vi "ReadSingleCANFrame.vi"(8 "error in (no error)":errorcluster, 11 "BLF File In":refnum<class "Read Write BLF.lvclass">) -> (0 "error out":errorcluster, 1 "CAN Channel":u16, 2 "CAN Frame":T1 {"type" items=["CAN Data"=0, "CAN Remote"=1, "CAN Bus Error"=2, "CAN 2.0 Data"=8, "CAN FD Data"=16, "CAN FD+BRS Data"=24, "J1939 Data"=192, "Delay"=224, "Log Trigger"=225, "Start Trigger"=226]; "payload" format="%x"; "timestamp" format="%<%.7X\n%x>T"; "identifier" format="%x"}, 3 "BLF File Out":refnum<class "Read Write BLF.lvclass">)   [LabVIEW 2015, in "Read Write BLF.lvclass"]
doc: "This VI will read <B>CAN Frames</B> from a BLF file. Optionally enter the <B>Offset</B> and <B>Length</B> which defaults to all. This will read the set number of Objects which might not correspond to the same number of frames.\n\n-------------\nBrian Hoover (Hooovahh)"
uses:
  Read Write BLF.lvclass
  Controls/Cluster - CAN Frame.ctl
  Controls/Enum - CAN Data Type.ctl
  Controls/Enum - Read Object Types.ctl
  Read Write BLF.lvclass/Read Write BLF.ctl
  SubVIs/GetBinlogdllpath.vi
  <vilib>/Utility/error.llb/Error Cluster From Error Code.vi
  <vilib>/Utility/libraryn.llb/Check if File or Folder Exists.vi
  <vilib>/Utility/file.llb/Application Directory.vi
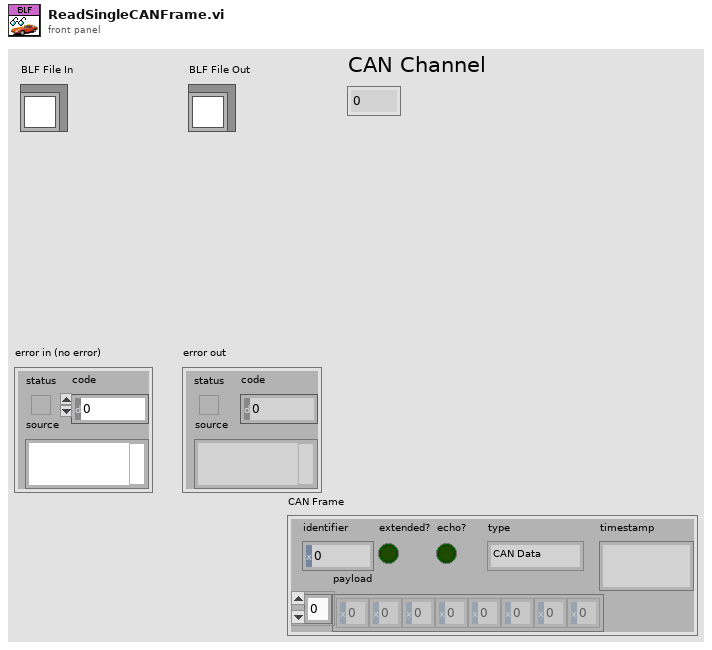
[diagram p1: front panel]
types:
  T1 = typedef "Read Write BLF.lvclass/Cluster - CAN Frame.ctl" = cluster{"timestamp":timestamp, "payload":u8[], "identifier":u32, "extended?":bool, "echo?":bool, "type":T2}
  T2 = typedef "Read Write BLF.lvclass/Enum - CAN Data Type.ctl" = u8
  T3 = typedef "Read Write BLF.lvclass/Enum - Read Object Types.ctl" = enum32{"UNKNOWN", "CAN_MESSAGE", "CAN_ERROR", "CAN_OVERLOAD", "CAN_STATISTIC", "APP_TRIGGER", "ENV_INTEGER", "ENV_DOUBLE", "ENV_STRING", "ENV_DATA", "LOG_CONTAINER", "LIN_MESSAGE", "LIN_CRC_ERROR", "LIN_DLC_INFO", "LIN_RCV_ERROR", "LIN_SND_ERROR", "LIN_SLV_TIMEOUT", "LIN_SCHED_MODCH", "LIN_SYN_ERROR", "LIN_BAUDRATE", "LIN_SLEEP", "LIN_WAKEUP", "MOST_SPY", "MOST_CTRL", "MOST_LIGHTLOCK", "MOST_STATISTIC", "reserved_1", "reserved_2", "reserved_3", "FLEXRAY_DATA", "FLEXRAY_SYNC", "CAN_DRIVER_ERROR", "MOST_PKT", "MOST_PKT2", "MOST_HWMODE", "MOST_REG", "MOST_GENREG", "MOST_NETSTATE", "MOST_DATALOST", "MOST_TRIGGER", "FLEXRAY_CYCLE", "FLEXRAY_MESSAGE", "LIN_CHECKSUM_INFO", "LIN_SPIKE_EVENT", "CAN_DRIVER_SYNC", "FLEXRAY_STATUS", "GPS_EVENT", "FR_ERROR", "FR_STATUS", "FR_STARTCYCLE", "FR_RCVMESSAGE", "REALTIMECLOCK", "AVAILABLE2", "AVAILABLE3", "LIN_STATISTIC", "J1708_MESSAGE", "J1708_VIRTUAL_MSG", "LIN_MESSAGE2", "LIN_SND_ERROR2", "LIN_SYN_ERROR2", "LIN_CRC_ERROR2", "LIN_RCV_ERROR2", "LIN_WAKEUP2", "LIN_SPIKE_EVENT2", "LIN_LONG_DOM_SIG", "APP_TEXT", "FR_RCVMESSAGE_EX", "MOST_STATISTICEX", "MOST_TXLIGHT", "MOST_ALLOCTAB", "MOST_STRESS", "ETHERNET_FRAME", "SYS_VARIABLE", "CAN_ERROR_EXT", "CAN_DRIVER_ERROR_EXT", "LIN_LONG_DOM_SIG2", "MOST_150_MESSAGE", "MOST_150_PKT", "MOST_ETHERNET_PKT", "MOST_150_MESSAGE_FRAGMENT", "MOST_150_PKT_FRAGMENT", "MOST_ETHERNET_PKT_FRAGMENT", "MOST_SYSTEM_EVENT", "MOST_150_ALLOCTAB", "MOST_50_MESSAGE", "MOST_50_PKT", "CAN_MESSAGE2", "LIN_UNEXPECTED_WAKEUP", "LIN_SHORT_OR_SLOW_RESPONSE", "LIN_DISTURBANCE_EVENT", "SERIAL_EVENT", "OVERRUN_ERROR", "EVENT_COMMENT", "WLAN_FRAME", "WLAN_STATISTIC", "MOST_ECL", "GLOBAL_MARKER", "AFDX_FRAME", "AFDX_STATISTIC", "KLINE_STATUSEVENT", "CAN_FD_MESSAGE", "CAN_FD_MESSAGE_64", "ETHERNET_RX_ERROR", "ETHERNET_STATUS", "CAN_FD_ERROR_64", "LIN_SHORT_OR_SLOW_RESPONSE2", "AFDX_STATUS", "AFDX_BUS_STATISTIC"}
  T4 = typedef "Read Write BLF.lvclass/Cluster - mHeaderBase.ctl" = cluster{"mSignature":u32, "mHeaderSize":u16, "mHeaderVersion":u16, "mObjectSize":u32, "Object Type":T3}
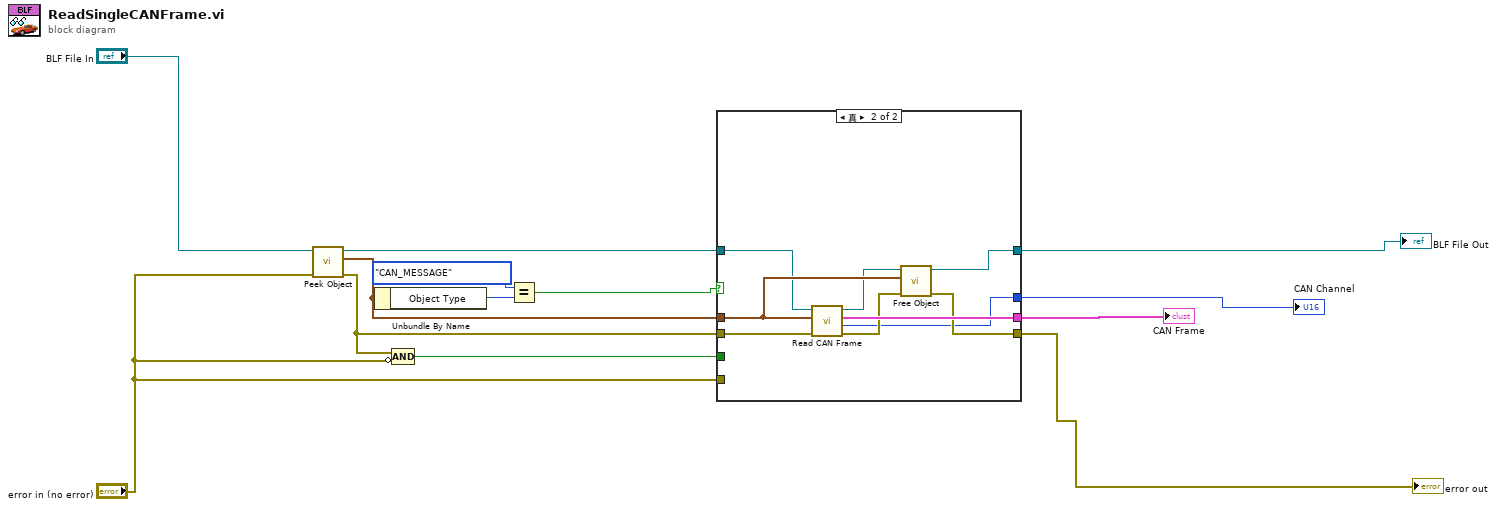
[diagram p0: block diagram]
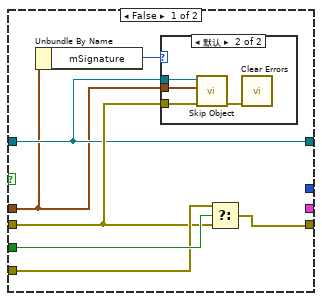
[diagram p2: hidden frame]
diagram:
  n1 = call "Peek Object.vi"("error in (no error)"="error in (no error)", "BLF File In"="BLF File In") -> ("error out"=w11:errorcluster, "Header Read"=w10:T4, "BLF File Out"=w12:refnum<class "Read Write BLF.lvclass">)  [unwired: 7 in]
  n2 = Unbundle By Name(w10) -> ("Object Type"=w5:T3)
  n3 = Compound Arithmetic op=AND(w11, invert "error in (no error)") -> (w13:bool)
  n4 = Equal?(x=Enum_-_Read_Object_Types."CAN_MESSAGE", y=w5) -> (x = y?=w6:bool)
  n5 = case shown="真" w6 {
    tunnel: [_ w33] -> w8
    tunnel: w12 -> [w16 w27]
    tunnel: [w16 w29] -> w9
    tunnel: w11 -> [w17 w32]
    tunnel: [w18 w30] -> w1
    tunnel: w10 -> [w15 w31]
    tunnel: w13 -> [w20 _]
    tunnel: "error in (no error)" -> [w19 _]
    tunnel: [_ w25] -> w7
    frame False {
      n6 = Unbundle By Name(w15) -> ("mSignature"=w14:u32)
      n7 = case shown="默认" w14 {
        tunnel: w17 -> [_ w24]
        tunnel: w16 -> [_ w22]
        tunnel: w15 -> [_ w21]
        frame 0 {
        }
        frame Default {
          n8 = call "Skip Object.vi"("error in (no error)"=w24, "Header"=w21, "BLF File In"=w22) -> ("error out"=w23:errorcluster)  [unwired: 7 in, 1 out]
          n9 = call <vilib>:"Clear Errors.vi"("error in (no error)"=w23) -> ()  [unwired: 5 in, 2 out]
        }
      }
      n10 = Select(t=w19, s=w20, f=w17) -> (s? t:f=w18:errorcluster)
    }
    frame True {
      n11 = call "Read CAN Frame.vi"("error in (no error)"=w32, "Header Read"=w31, "BLF File In"=w27) -> ("error out"=w28:errorcluster, "CAN Channel"=w25:u16, "CAN Frame"=w33:T1, "BLF File Out"=w26:refnum<class "Read Write BLF.lvclass">)  [unwired: 5 in]
      n12 = call "Free Object.vi"("error in (no error)"=w28, "Header"=w31, "BLF File In"=w26) -> ("error out"=w30:errorcluster, "BLF File Out"=w29:refnum<class "Read Write BLF.lvclass">)  [unwired: 7 in]
    }
  }
  "error out" <- w1
  "BLF File Out" <- w9
  "CAN Frame" <- w8
  "CAN Channel" <- w7
